vi "Field Delete From Array.vi"(10 "Field ID to Delete (\"\")":string, 11 "Field Array":T1[](array[typedef])) -> (2 "Index":i32, 3 "Field Array Out":T1[](array[typedef]))   [LabVIEW 2011]
uses:
  Field Record.ctl
  Field DataTypes.ctl
  Field NextItem.ctl
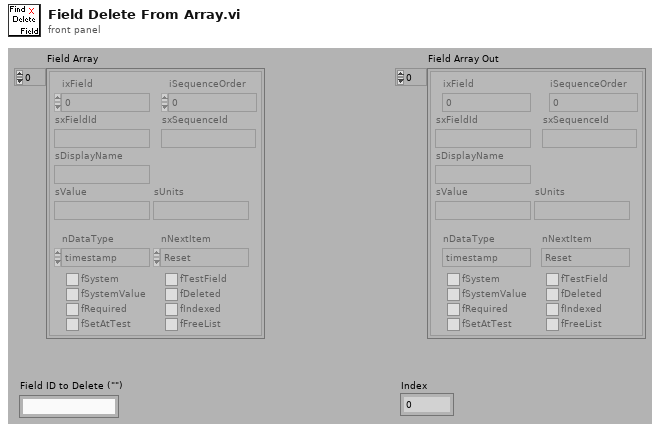
[diagram p1: front panel]
types:
  T1 = typedef "Field Record.ctl" = cluster{"ixField":i32, "iSequenceOrder":i32, "sxFieldId":string, "sxSequenceId":string, "sDisplayName":string, "sValue":string, "sUnits":string, "nDataType":T2, "nNextItem":T3, "fSystem":bool, "fSystemValue":bool, "fRequired":bool, "fSetAtTest":bool, "fTestField":bool, "fDeleted":bool, "fIndexed":bool, "fFreeList":bool}
  T2 = typedef "Field DataTypes.ctl" = enum32{"text", "numeric", "list", "timestamp", "boolean"}
  T3 = typedef "Field NextItem.ctl" = enum32{"Reset", "Retain", "Auto-Increment"}
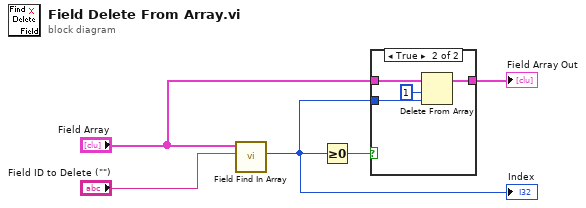
[diagram p0: block diagram]
diagram:
  n1 = call "Field Find In Array.vi"("FieldID or Display Name(\"\")"="Field ID to Delete (\"\")", "Field Array"="Field Array") -> ("Index"=w1:i32)  [unwired: 1 in, 8 out]
  "Index" <- w1
  n2 = Greater Or Equal To 0?(x=w1) -> (x >= 0?=w2:bool)
  n3 = case shown="True" w2 {
    tunnel: "Field Array" -> [w6 w10]
    tunnel: [w6 w9] -> w5
    tunnel: w1 -> [_ w8]
    frame False {
    }
    frame True {
      n4 = Delete From Array(array=w10, length=1, index=w8) -> (array with subset deleted=w9:T1[])  [unwired: 1 out]
    }
  }
  "Field Array Out" <- w5
